vi "Create and Add Instruments.vi"(6 "Physical Instr CFGs":string[](array[string]), 8 "error in":errorcluster, 11 "Target MSS in":refnum<class "MSS Target Actor.lvclass">) -> (0 "error out":errorcluster, 3 "Target MSS out":refnum<class "MSS Target Actor.lvclass">)   [LabVIEW 2023]
uses:
  MSS Target Actor.lvclass/MSS Target Actor.ctl
  Target Measure and Stimulus Subsystems.lvclass
  MSS Target Actor.lvclass
  C:/Program Files/National Instruments/LabVIEW 2023/vi.lib/ActorFramework/Actor/Actor.lvclass
  D:/git/HAL/HAL GOOP4/Target Measure and Stimulus Subsystems/Target Measure and Stimulus Subsystems/MSS Target Actor.lvclass
  D:/git/HAL/HAL GOOP4/Target Measure and Stimulus Subsystems/IMSS Target Actor/IMSS Target Actor.lvclass
  C:/Program Files/National Instruments/LabVIEW 2023/vi.lib/ni/Actors/Network Endpoint Actors/Nested Endpoint Caller/Nested Endpoint Caller/Nested Endpoint Caller.lvclass
  D:/git/HAL/HAL GOOP4/Host Measure and Stimulus Subsystems/Host Measure and Stimulus Subsystems.lvclass
  D:/git/HAL/HAL GOOP4/Target Measure and Stimulus Subsystems/Target Measure and Stimulus Subsystems.lvclass
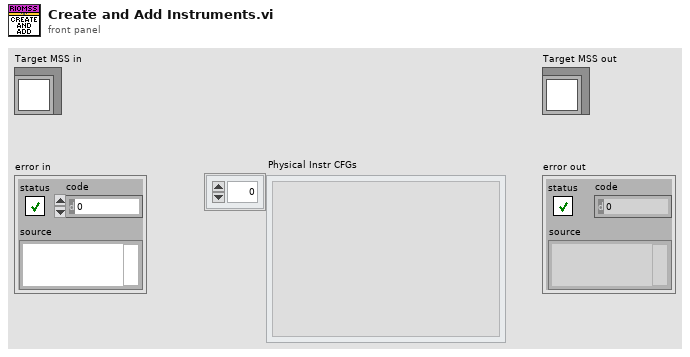
[diagram p1: front panel]
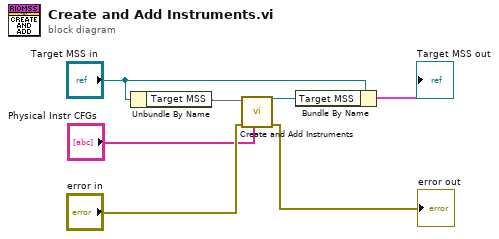
[diagram p0: block diagram]
diagram:
  n1 = Unbundle By Name("Target MSS in") -> ("Target MSS"=w6)
  n2 = call-dynamic "Create and Add Instruments.vi"("Physical Instr CFGs"="Physical Instr CFGs", "Error In"="error in", "Target Measure and Stimulus Subsystems in"=w6) -> ("Error Out"=→"error out":errorcluster, "Target Measure and Stimulus Subsystems out"=w2:refnum<class "Target Measure and Stimulus Subsystems.lvclass">)  [unwired: 7 in]
  n3 = Bundle By Name(cluster="Target MSS in", "Target MSS"=w2) -> (→"Target MSS out":cluster{})
